vi "kAverager.vi"(8 "num avg":i32=10, 11 "input":dbl) -> (3 "output":dbl)   [LabVIEW 2018, in "kevLib2011.lvlib"]
uses:
  kevLib2011.lvlib
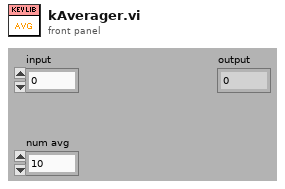
[diagram p1: front panel]
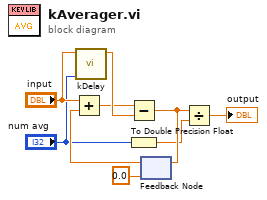
[diagram p0: block diagram]
diagram:
  n1 = call "kDelay.vi"("delay"="num avg", "input"="input") -> ("output"=w8:dbl)  [unwired: 9 in]
  n2 = To Double Precision Float(number="num avg") -> (double precision float=w2:dbl)
  n3 = feedback #1(0.0) -> (w6:dbl)
  n4 = Add(x="input", y=w6) -> (x+y=w7:dbl)
  n5 = Subtract(x=w7, y=w8) -> (x-y=w4:dbl)
  n6 = feedback-in #1(w4) -> ()
  n7 = Divide(x=w4, y=w2) -> (x/y=→"output":dbl)
